vi "Begin.vi"(11 "Image Size":T1=enum."160x120") -> (0 "error out":errorcluster)   [LabVIEW 2012]
doc: "Called before other user functions, this VI is expected to open initial I/O refnums, load in file data, and do all program initialization. Notice that the <B>error out</B> terminal is simply used for data flow. Wiring it to other structures or subVIs ensures that this VI runs first."
uses:
  <vilib>/Rock Robotics/WPI/Camera/WPI_CameraImageSize.ctl
  <vilib>/Rock Robotics/WPI/Camera/WPI_CameraWhite Balance Values.ctl
  <vilib>/Rock Robotics/WPI/Camera/WPI_CameraExposure Values.ctl
  <vilib>/Rock Robotics/WPI/Camera/WPI_CameraFrameRate.ctl
  <vilib>/Rock Robotics/WPI/DriverStation/WPI_DriverStationRobotMode2.ctl
  <vilib>/Rock Robotics/WPI/Joystick/WPI_JoystickDeviceEnum.ctl
  <vilib>/Rock Robotics/SystemInterfaces/DIO/FPGA_DIOPWMChannel.ctl
  <vilib>/Rock Robotics/WPI/SafetyOutput/WPI_SafetyOutputConfigMenu.ctl
  <vilib>/Rock Robotics/SystemInterfaces/DIO/FPGA_DIORelayChannel.ctl
  <vilib>/Rock Robotics/SystemInterfaces/DIO/FPGA_DIOChannel.ctl
  Robot Global Data.vi
  <vilib>/Rock Robotics/WPI/RobotDrive/WPI_RobotDriveOpen4MotorWithVictor.vi
  <vilib>/Rock Robotics/WPI/MotorControl/WPI_MotorControlOpen Victor.vi
  <vilib>/Rock Robotics/WPI/Compressor/WPI_CompressorGetSetRefNum.vi
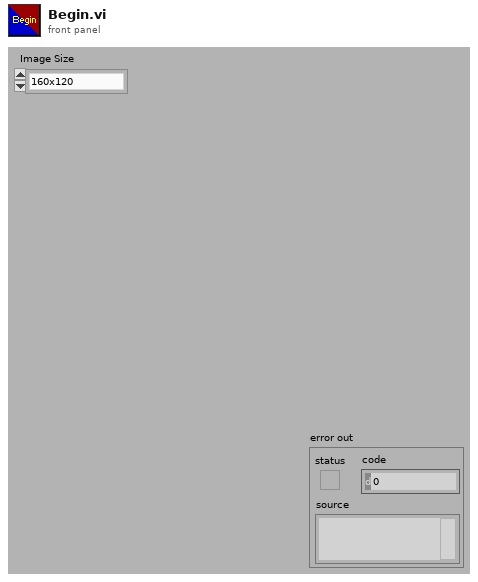
[diagram p1: front panel]
types:
  T1 = typedef "WPI_CameraImageSize.ctl" = enum16{"640x480", "320x240", "160x120"}
  T2 = typedef "FPGA_DIORelayChannel.ctl" = enum8{"Relay 1", "Relay 2", "Relay 3", "Relay 4", "Relay 5", "Relay 6", "Relay 7", "Relay 8", "Invalid"}
  T3 = typedef "FPGA_DIOChannel.ctl" = enum8{"DIO 1", "DIO 2", "DIO 3", "DIO 4", "DIO 5", "DIO 6", "DIO 7", "DIO 8", "DIO 9", "DIO 10", "DIO 11", "DIO 12", "DIO 13", "DIO 14", "Invalid"}
  T4 = typedef "FPGA_DIOPWMChannel.ctl" = enum8{"PWM 1", "PWM 2", "PWM 3", "PWM 4", "PWM 5", "PWM 6", "PWM 7", "PWM 8", "PWM 9", "PWM 10", "Invalid"}
  T5 = typedef "WPI_SafetyOutputConfigMenu.ctl" = enum16{"Enable", "Disable"}
  T6 = typedef "WPI_JoystickDeviceEnum.ctl" = enum16{"USB 1", "USB 2", "USB 3", "USB 4", "Kinect 1", "Kinect 2"}
  T7 = typedef "WPI_DriverStationRobotMode2.ctl" = enum16{"Autonomous Disabled", "Autonomous Enabled", "Teleop Disabled", "Teleop Enabled", "Timeout", "Finish", "Test Disabled", "Test Enabled"}
  T8 = typedef "WPI_CameraFrameRate.ctl" = u32
  T9 = typedef "WPI_CameraExposure Values.ctl" = enum16{"Auto", "Flicker-free 50 Hz", "Flicker-free 60 Hz", "Hold current"}
  T10 = typedef "WPI_CameraWhite Balance Values.ctl" = enum16{"Auto", "Fixed indoor", "Fixed outdoor 1", "Fixed outdoor 2", "Fixed fluorescent 1", "Fixed fluorescent 2", "Hold current"}
  T11 = typedef "WPI_RobotDriveDevRef.ctl" = cluster{"DevStatus":errorcluster, "Motors[]":T12[], "Square Inputs":bool, "Max Output":dbl, "Isochronous":bool}
  T12 = typedef "WPI_MotorControlDeviceRef.ctl" = cluster{"DeviceStatus":errorcluster, "Type":enum16{"PWM", "CAN"}, "PWM":cluster{"Digital Module":T13, "PWM Channel":T4, "DeadBand":T14}, "CAN":cluster{"Device Number":u8, "Control Mode":T15, "Semaphore":T16, "Max Vout":dbl}, "Invert":bool, "TransformRef":T17, "InvTransformRef":T17}
  T13 = typedef "FPGA_TypedefDigitalModule.ctl" = enum16{"Digital Module 1", "Digital Module 2"}
  T14 = typedef "WPI_PWMDeadband.ctl" = cluster{"Name":string, "maxPositivePwm":i32, "minPositivePwm":i32, "centerPwm":i32, "maxNegativePwm":i32, "minNegativePwm":i32, "angularRange":u16}
  T15 = typedef "WPI_CANJaguar_ControlMode.ctl" = enum8{"Percent VBus", "Current", "Speed", "Position", "Voltage"}
  T16 = typedef "Semaphore RefNum" = refnum<k1>
  T17 = typedef "WPI_PWMTransform_ConPane.ctl" = refnum<vi>
  T18 = typedef "WPI_CameraDevRef.ctl" = cluster{"Camera Address":string, "CameraStatus":errorcluster, "Acquire Image Notifier":refnum<notifier>}
  T19 = typedef "WPI_JoystickDevRef.ctl" = cluster{"Device":T6}
  T20 = typedef "WPI_RelayDevRef.ctl" = cluster{"DevStatus":errorcluster, "Relay Channel":T2, "Digital Module":T13, "Relay Direction":T21}
  T21 = typedef "WPI_RelayDirection.ctl" = enum16{"Both directions", "Forward only", "Reverse only"}
  T22 = typedef "WPI_CompressorDevRef.ctl" = cluster{"DevStatus":errorcluster, "DigitalInputDevRef":T23, "RelayDevRef":T20}
  T23 = typedef "WPI_DigitalInputDevRef.ctl" = cluster{"DevStatus":errorcluster, "DIO Channel":T3, "Digital Module":T13}
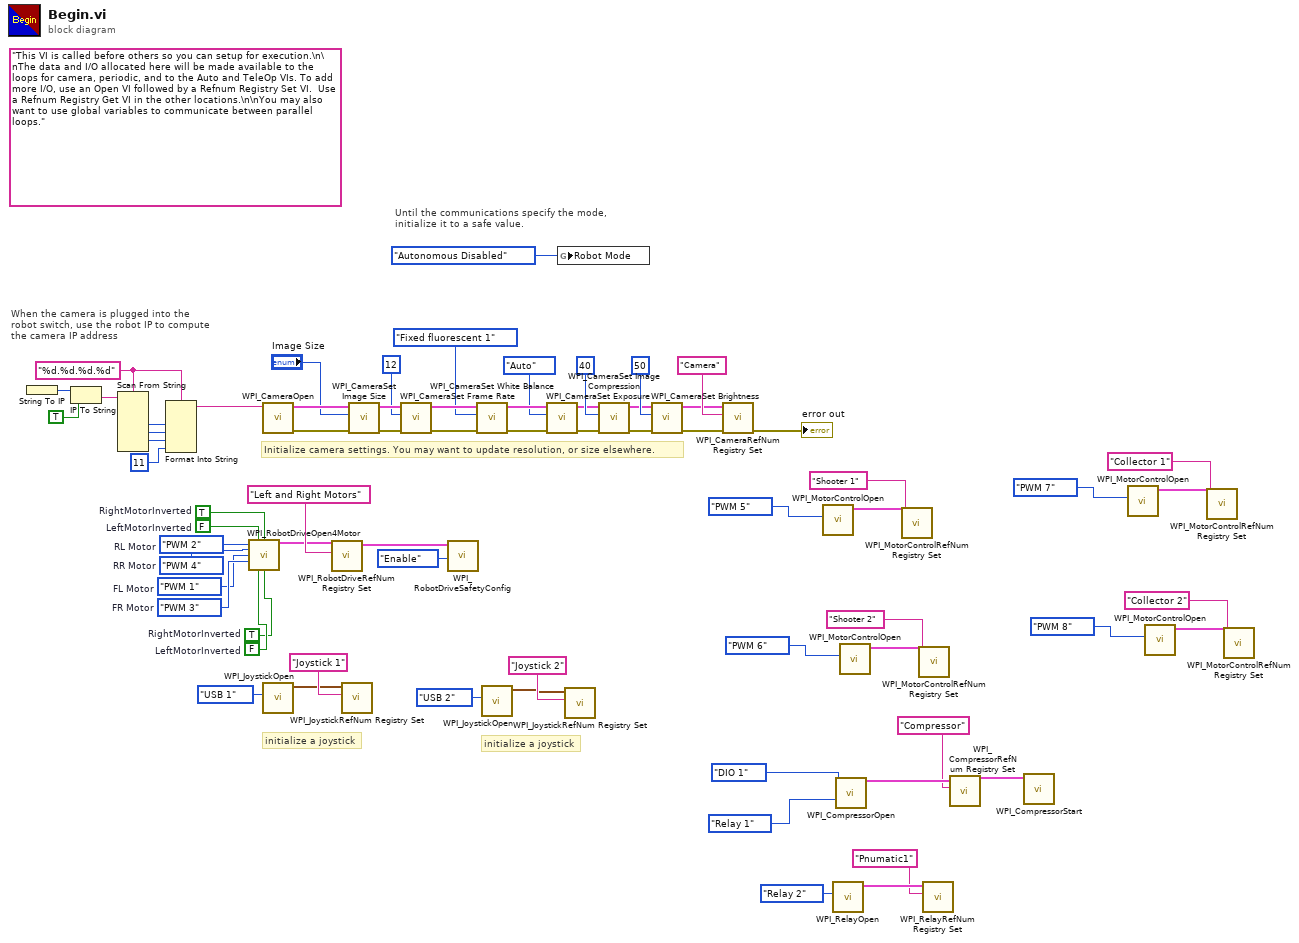
[diagram p0: block diagram]
diagram:
  w22 = FALSE  # LeftMotorInverted
  w21 = TRUE  # RightMotorInverted
  w29 = FPGA_DIOPWMChannel."PWM 3"  # FR Motor
  w28 = FPGA_DIOPWMChannel."PWM 1"  # FL Motor
  w27 = FPGA_DIOPWMChannel."PWM 4"  # RR Motor
  w26 = FPGA_DIOPWMChannel."PWM 2"  # RL Motor
  w25 = FALSE  # LeftMotorInverted
  w24 = TRUE  # RightMotorInverted
  w42 = "%d.%d.%d.%d" ("format string")
  (unwired) "This VI is called before others so you can setup for execution.\n\nThe data and I/O allocated here will be made available to the loops for camera, periodic, and to the Auto and TeleOp VIs. To add more I/O, use an Open VI followed by a Refnum Registry Set VI.  Use a Refnum Registry Get VI in the other locations.\n\nYou may also want to use global variables to communicate between parallel loops."
  # "initialize a joystick"
  # "initialize a joystick"
  # "Until the communications specify the mode,\ninitialize it to a safe value."
  # "When the camera is plugged into the\nrobot switch, use the robot IP to compute\nthe camera IP address"
  # "Initialize camera settings. You may want to update resolution, or size elsewhere."
  n1 = String To IP() -> (0:w49:u32)  [unwired: 1 in]
  n2 = IP To String(1:TRUE ("dot notation? (F)"), 2:w49) -> (0:w47:string)
  n3 = Scan From String(format string=w42, input string=w47) -> (output 1=w46:i32, output 2=w45:i32, output 3=w44:i32)  [unwired: 7 in, 3 out]
  n4 = Format Into String(format string=w42, w46, w45, w44, 11 ("Compression")) -> (resulting string=w40:string)  [unwired: 2 in, 1 out]
  n5 = call-poly <vilib>:"WPI_RobotDriveOpen4Motor.vi"("Rear Left Motor"=w26, "Rear Left Motor Inverted"=w25, "Rear Right Motor Inverted"=w24, "Rear Right Motor"=w27, "Front Left Motor"=w28, "Front Right Motor"=w29, "Front Left Motor Inverted"=w22, "Front Right Motor Inverted"=w21) -> ("RobotDriveDevRef"=w23:T11)  [unwired: 6 in, 1 out]
  n6 = call <vilib>:"WPI_CameraOpen.vi"("Camera Address"=w40) -> ("error out"=w61:errorcluster, "CameraDevRef"=w62:T18)  [unwired: 1 in, 8 out]
  n7 = call <vilib>:"WPI_JoystickOpen.vi"("JoystickDevice"=WPI_JoystickDeviceEnum."USB 1") -> ("JoystickDevRef"=w38:T19)  [unwired: 10 in]
  n8 = call <vilib>:"WPI_RobotDriveRefNum Registry Set.vi"("refnum name"="Left and Right Motors", "RobotDriveDevRef"=w23) -> ("RobotDriveDevRef"=w31:T11)  [unwired: 1 in, 8 out]
  n9 = call <vilib>:"WPI_JoystickRefNum Registry Set.vi"("refnum name"="Joystick 1", "JoystickDevRef"=w38) -> ()  [unwired: 8 in, 2 out]
  n10 = call <vilib>:"WPI_CameraSet Image Size.vi"("error in (no error)"=w61, "Image Size"="Image Size", "CameraDevRef"=w62) -> ("error out"=w60:errorcluster, "CameraDevRef Out"=w63:T18)  [unwired: 7 out]
  n11 = call <vilib>:"WPI_CameraSet Frame Rate.vi"("error in (no error)"=w60, "Frame Rate (fps)"=T8 12, "CameraDevRef"=w63) -> ("error out"=w59:errorcluster, "CameraDevRef Out"=w65:T18)  [unwired: 7 out]
  n12 = call <vilib>:"WPI_RobotDriveSafetyConfig.vi"("mode"=WPI_SafetyOutputConfigMenu."Enable", "RobotDriveDevRef"=w31) -> ()  [unwired: 8 in, 2 out]
  n13 = call <vilib>:"WPI_CameraSet White Balance.vi"("error in (no error)"=w59, "White Balance"=WPI_CameraWhite_Balance_Values."Fixed fluorescent 1", "CameraDevRef"=w65) -> ("error out"=w58:errorcluster, "CameraDevRef Out"=w64:T18)  [unwired: 7 out]
  n14 = call <vilib>:"WPI_JoystickOpen.vi"("JoystickDevice"=WPI_JoystickDeviceEnum."USB 2") -> ("JoystickDevRef"=w34:T19)  [unwired: 10 in]
  n15 = call <vilib>:"WPI_CameraSet Exposure.vi"("error in (no error)"=w58, "Exposure"=WPI_CameraExposure_Values."Auto", "CameraDevRef"=w64) -> ("error out"=w57:errorcluster, "CameraDevRef Out"=w67:T18)  [unwired: 7 out]
  n16 = global write "Robot Global Data.vi" "Robot Mode"(WPI_DriverStationRobotMode2."Autonomous Disabled" ("Robot Mode")) -> ()
  n17 = call <vilib>:"WPI_JoystickRefNum Registry Set.vi"("refnum name"="Joystick 2", "JoystickDevRef"=w34) -> ()  [unwired: 8 in, 2 out]
  n18 = call <vilib>:"WPI_CameraSet Image Compression.vi"("error in (no error)"=w57, "Compression"=40, "CameraDevRef"=w67) -> ("error out"=w56:errorcluster, "CameraDevRef Out"=w66:T18)  [unwired: 7 out]
  n19 = call <vilib>:"WPI_CameraSet Brightness.vi"("error in (no error)"=w56, "Brightness"=50, "CameraDevRef"=w66) -> ("error out"=w54:errorcluster, "CameraDevRef Out"=w55:T18)  [unwired: 7 out]
  n20 = call <vilib>:"WPI_CameraRefNum Registry Set.vi"("error in (no error)"=w54, "refnum name"="Camera", "CameraDevRef"=w55) -> ("error out"=→"error out":errorcluster)  [unwired: 8 out]
  n21 = call-poly <vilib>:"WPI_MotorControlOpen.vi"("PWM Channel"=FPGA_DIOPWMChannel."PWM 5") -> ("MotorControlDeviceRef"=w20:T12)  [unwired: 9 in, 1 out]
  n22 = call <vilib>:"WPI_RelayOpen.vi"("Relay Channel"=FPGA_DIORelayChannel."Relay 2") -> ("RelayDevRef"=w3:T20)  [unwired: 9 in, 1 out]
  n23 = call <vilib>:"WPI_CompressorOpen.vi"("Pressure Switch DIO Channel"=FPGA_DIOChannel."DIO 1", "Relay Channel"=FPGA_DIORelayChannel."Relay 1") -> ("CompressorDevRef"=w7:T22)  [unwired: 12 in, 1 out]
  n24 = call-poly <vilib>:"WPI_MotorControlOpen.vi"("PWM Channel"=FPGA_DIOPWMChannel."PWM 6") -> ("MotorControlDeviceRef"=w18:T12)  [unwired: 9 in, 1 out]
  n25 = call <vilib>:"WPI_MotorControlRefNum Registry Set.vi"("refnum name"="Shooter 1", "MotorControlDevRef"=w20) -> ()  [unwired: 8 in, 2 out]
  n26 = call <vilib>:"WPI_MotorControlRefNum Registry Set.vi"("refnum name"="Shooter 2", "MotorControlDevRef"=w18) -> ()  [unwired: 8 in, 2 out]
  n27 = call <vilib>:"WPI_RelayRefNum Registry Set.vi"("refnum name"="Pnumatic1", "RelayDevRef"=w3) -> ()  [unwired: 8 in, 2 out]
  n28 = call <vilib>:"WPI_CompressorRefNum Registry Set.vi"("refnum name"="Compressor", "CompressorDevRef"=w7) -> ("CompressorDevRef"=w5:T22)  [unwired: 8 in, 1 out]
  n29 = call <vilib>:"WPI_CompressorStart.vi"("CompressorDevRef"=w5) -> ()  [unwired: 9 in, 2 out]
  n30 = call-poly <vilib>:"WPI_MotorControlOpen.vi"("PWM Channel"=FPGA_DIOPWMChannel."PWM 7") -> ("MotorControlDeviceRef"=w15:T12)  [unwired: 9 in, 1 out]
  n31 = call-poly <vilib>:"WPI_MotorControlOpen.vi"("PWM Channel"=FPGA_DIOPWMChannel."PWM 8") -> ("MotorControlDeviceRef"=w12:T12)  [unwired: 9 in, 1 out]
  n32 = call <vilib>:"WPI_MotorControlRefNum Registry Set.vi"("refnum name"="Collector 1", "MotorControlDevRef"=w15) -> ()  [unwired: 8 in, 2 out]
  n33 = call <vilib>:"WPI_MotorControlRefNum Registry Set.vi"("refnum name"="Collector 2", "MotorControlDevRef"=w12) -> ()  [unwired: 8 in, 2 out]
